vi "UI Set Chart DisableState.vi"(7 "Enable?":bool=TRUE, 8 "error in (no error)":errorcluster, 11 "UI.Chart.Refs":T1) -> (0 "error out":errorcluster, 3 "UI.Chart.Refs":T1)   [LabVIEW 2019, in "Control Workspace Shared.lvlib"]
uses:
  Types/UI.Chart.Refs.ctl
  Control Workspace Shared.lvlib
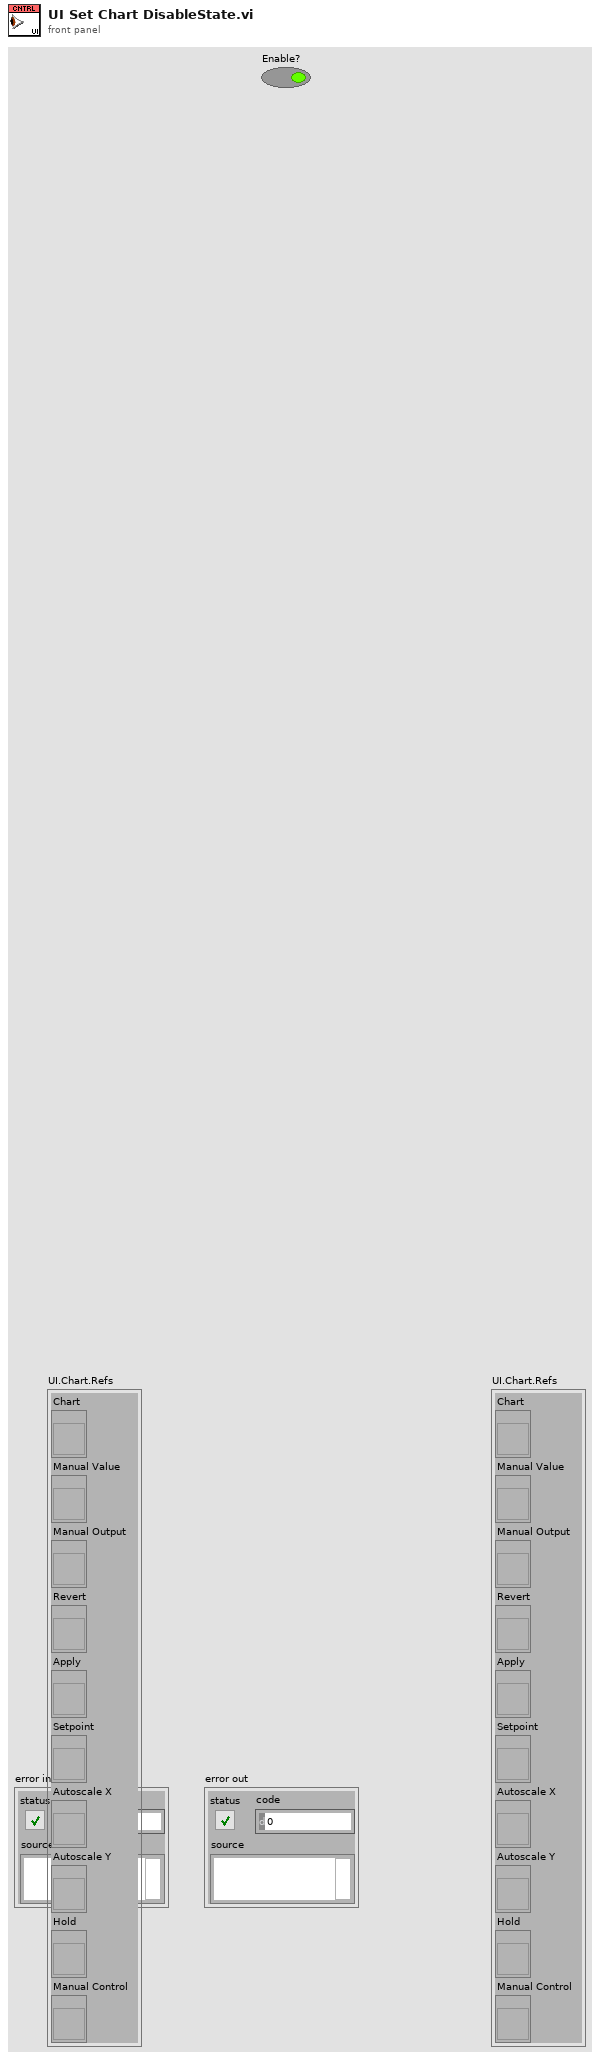
[diagram p1: front panel]
types:
  T1 = typedef "Control Workspace Shared.lvlib/UI.Chart.Refs.ctl" = cluster{"Chart":refnum<vi>, "Manual Value":refnum<vi>, "Manual Output":refnum<vi>, "Revert":refnum<vi>, "Apply":refnum<vi>, "Setpoint":refnum<vi>, "Autoscale X":refnum<vi>, "Autoscale Y":refnum<vi>, "Hold":refnum<vi>, "Manual Control":refnum<vi>}
  T2 = enum8{"Enabled", "Disabled", "Disabled and Grayed Out"}
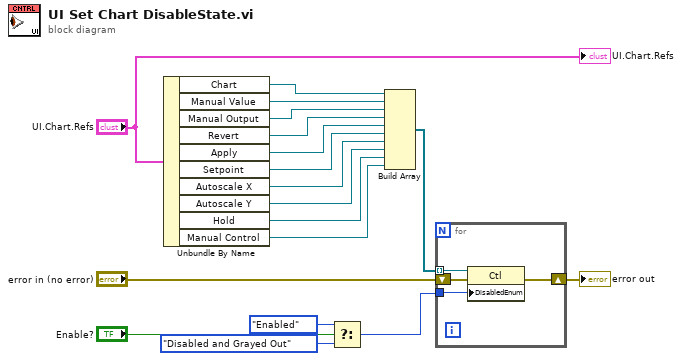
[diagram p0: block diagram]
diagram:
  n1 = Unbundle By Name("UI.Chart.Refs") -> ("Chart"=w18:refnum<vi>, "Manual Value"=w17:refnum<vi>, "Manual Output"=w16:refnum<vi>, "Revert"=w15:refnum<vi>, "Apply"=w14:refnum<vi>, "Setpoint"=w13:refnum<vi>, "Autoscale X"=w4:refnum<vi>, "Autoscale Y"=w3:refnum<vi>, "Hold"=w2:refnum<vi>, "Manual Control"=w1:refnum<vi>)
  n2 = Select(t=T2."Enabled" ("Disabled"), s="Enable?", f=T2."Disabled and Grayed Out" ("Disabled")) -> (s? t:f=w5:T2)
  n3 = Build Array(w18, w17, w16, w15, w14, w13, w4, w3, w2, w1) -> (w12:refnum<vi>[])
  n4 = for {
    tunnel: w12 -> [w22] mode=indexing
    shift-right: [w20] -> w10
    shift-left: "error in (no error)" -> [w21]
    tunnel: w5 -> [w19]
    n5 = property class="Ctl"(reference=w22, error in=w21, "DisabledEnum"=w19) -> (error out=w20:errorcluster)  [unwired: 1 out]
  }
  "error out" <- w10
  "UI.Chart.Refs" <- "UI.Chart.Refs"
